vi "mtg - save file.vi"(7 "hourly file?":bool, 9 "history data":dbl[][](array[numeric]), 10 "date time info":T1) -> ()   [LabVIEW 2025]
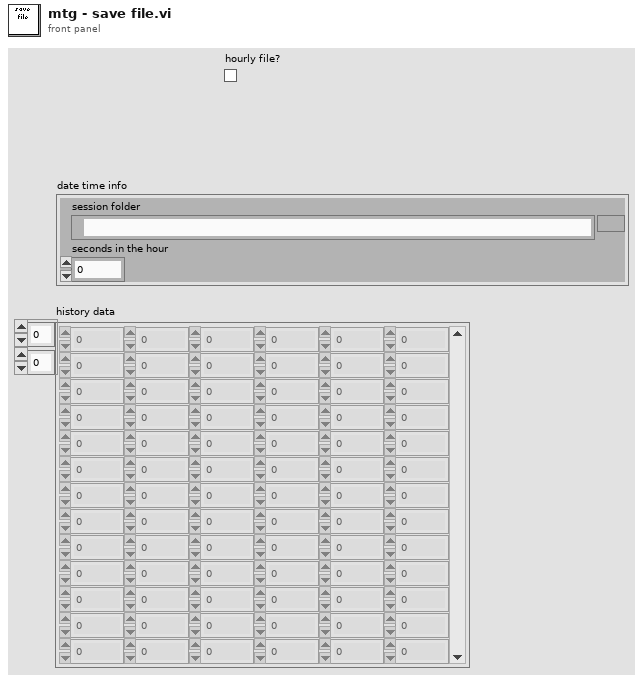
[diagram p1: front panel]
types:
  T1 = cluster{"session folder":path, "seconds in the hour":i32}
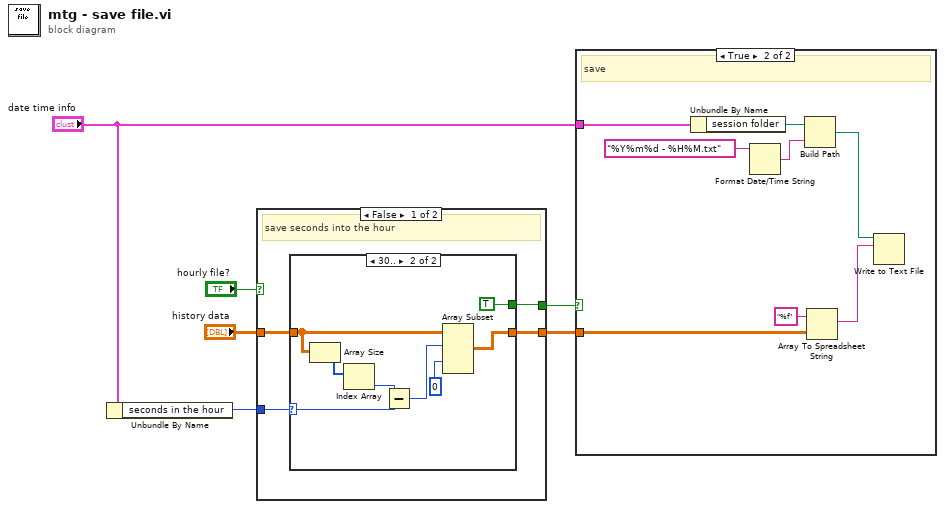
[diagram p0: block diagram]
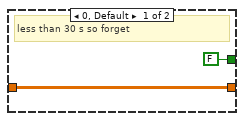
[diagram p3: hidden frame]
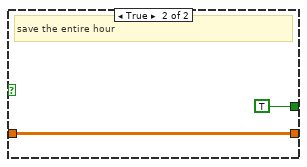
[diagram p4: hidden frame]
diagram:
  n1 = Unbundle By Name("date time info") -> ("seconds in the hour"=w2:i32)
  n2 = case shown="False" "hourly file?" {
    tunnel: "history data" -> [w10 w22]
    tunnel: [w9 w22] -> w4
    tunnel: w2 -> [w8 _]
    tunnel: [w7 TRUE] -> w1
    frame False {
      # "save seconds into the hour"
      n3 = case shown="30.." w8 {
        selector: w8 -> [_ w17]
        tunnel: w10 -> [w11 w15]
        tunnel: [w11 w20] -> w9
        tunnel: [FALSE TRUE] -> w7
        frame 0, Default {
          # "less than 30 s so forget"
        }
        frame 30.. {
          n4 = Array Size(array=w15) -> (size(s)=w14:i32[])
          n5 = Index Array(array=w14) -> (element=w13:i32)  [unwired: 1 in]
          n6 = Subtract(x=w13, y=w17) -> (x-y=w19:i32)
          n7 = Array Subset(array=w15, index (row)=w19, index (col)=0 ("index")) -> (w20:dbl[][])  [unwired: 2 in]
        }
      }
    }
    frame True {
      # "save the entire hour"
    }
  }
  n8 = case shown="True" w1 {
    tunnel: w4 -> [_ w26]
    tunnel: "date time info" -> [_ w25]
    frame False {
      # "forget"
    }
    frame True {
      # "save"
      n9 = Unbundle By Name(w25) -> ("session folder"=w24:path)
      n10 = Format Date/Time String(time format string (%c)="%Y%m%d - %H%M.txt") -> (date/time string=w29:string)  [unwired: 2 in]
      n11 = Build Path(base path=w24, name or relative path=w29) -> (appended path=w30:path)
      n12 = Array To Spreadsheet String(array=w26, 3:"%f" ("format string")) -> (spreadsheet string=w23:string)  [unwired: 1 in]
      n13 = Write to Text File(file (use dialog)=w30, text=w23) -> ()  [unwired: 2 in, 3 out]
    }
  }
